vi "Get Map Image Path.vi"(1 "name or relative path":string="/images/BlueTeam.jpg") -> (0 "Image Path":path)   [LabVIEW 2012]
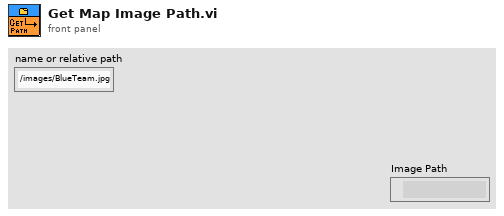
[diagram p1: front panel]
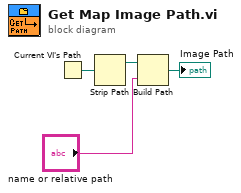
[diagram p0: block diagram]
diagram:
  n1 = Current VI's Path() -> (path=w4:path)
  n2 = Strip Path(path=w4) -> (stripped path=w3:path)  [unwired: 1 out]
  n3 = Build Path(base path=w3, name or relative path="name or relative path") -> (appended path=→"Image Path":path)
